vi "Remote APIs for base station configuration Action Command.vi"(8 "error in (no error)":errorcluster, 9 "Command":string, 10 "Cellular Technology":T1, 11 "Base Station":T2) -> (0 "error out":errorcluster)   [LabVIEW 2021]
uses:
  Controls/TCP_FGV.ctl
  Controls/Base_Station_Emulator.ctl
  Controls/Cellular_Technology.ctl
panel:
  out "Output String":string
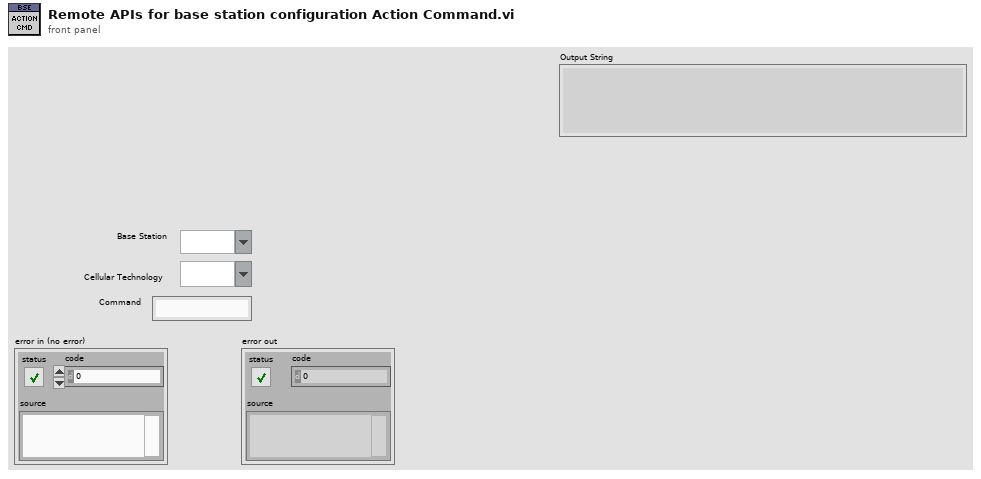
[diagram p1: front panel]
types:
  T1 = typedef "Cellular_Technology.ctl" = string
  T2 = typedef "Base_Station_Emulator.ctl" = string
  T3 = typedef "TCP_FGV.ctl" = enum16{"Open", "Read", "Write", "Close"}
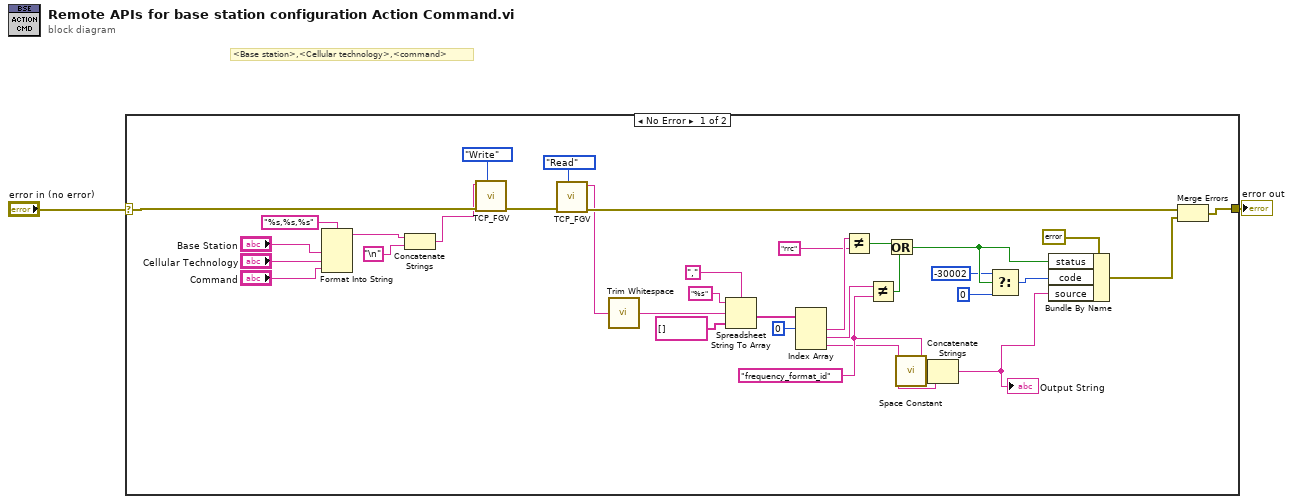
[diagram p0: block diagram]
diagram:
  # "<Base station>,<Cellular technology>,<command>"
  n1 = case shown="No Error" "error in (no error)" {
    selector: "error in (no error)" -> [w32 w38]
    tunnel: [w3 w38] -> w1
    frame No Error {
      w9 = "frequency_format_id"
      n2 = Format Into String(format string="%s,%s,%s", "Base Station", "Cellular Technology", "Command") -> (resulting string=w30:string)  [unwired: 2 in, 1 out]
      n3 = Concatenate Strings(w30, "\n") -> (w29:string)
      n4 = call "TCP_FGV.vi"("Command"=w29, "error in (no error)"=w32, "Operation"=TCP_FGV."Write") -> ("error out"=w4:errorcluster)  [unwired: 6 in, 1 out]
      n5 = call "TCP_FGV.vi"("error in (no error)"=w4, "Operation"=TCP_FGV."Read") -> ("Data Out"=w6:string, "error out"=w12:errorcluster)  [unwired: 7 in]
      n6 = call <vilib>:"Trim Whitespace.vi"("string"=w6) -> ("trimmed string"=w26:string)  [unwired: 1 in]
      n7 = Spreadsheet String To Array(delimiter (Tab)=",", format string="%s", spreadsheet string=w26, array type (2D Dbl)=string[] []) -> (array=w22:string[])
      n8 = Index Array(array=w22, index #1=0 ("index")) -> (element #1=w23:string, element #2=w13:string, element #3=w8:string)  [unwired: 2 in]
      n9 = Not Equal?(x=w23, y="rrc" ("format string")) -> (x != y?=w24:bool)
      n10 = Not Equal?(x=w13, y=w9) -> (x != y?=w25:bool)
      n11 = Or(x=w24, y=w25) -> (x .or. y?=w27:bool)
      n12 = call <vilib>:"Space Constant.vi"() -> ("String"=w10:string)
      n13 = Concatenate Strings(w9, w10, w8) -> (w7:string)
      "Output String" <- w7
      n14 = Select(t=-30002 ("code"), s=w27, f=0 ("code")) -> (s? t:f=w28:i32)
      n15 = Bundle By Name(cluster=errorcluster {"status"=FALSE, "code"=0, "source"=""} ("error constant"), "status"=w27, "code"=w28, "source"=w7) -> (w11:errorcluster)
      n16 = Merge Errors(w12, w11) -> (w3:errorcluster)
    }
    frame Error {
    }
  }
  "error out" <- w1
